vi "Set Image Size.vi"(8 "error in (no error)":errorcluster caption="错误输入（无错误）", 9 "Height":i32, 10 "Width":i32, 11 "ImageListClass 输入":refnum<class "ImageListClass.lvclass"> caption="DNL_LabVIEW Object in") -> (0 "error out":errorcluster caption="错误输出", 3 "ImageListClass 输出":refnum<class "ImageListClass.lvclass"> caption="DNL_LabVIEW Object out")   [LabVIEW 2013, in "ImageListClass.lvclass"]
uses:
  ImageListClass.lvclass
  ImageListClass.lvclass/ImageListClass.ctl
  System.Drawing
  System.Windows.Forms
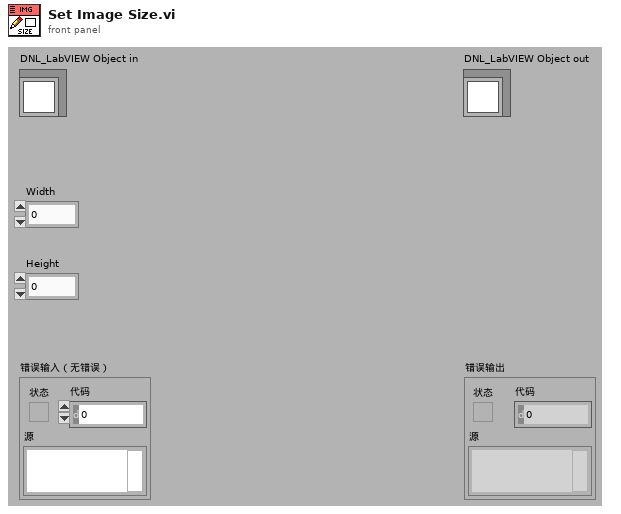
[diagram p1: front panel]
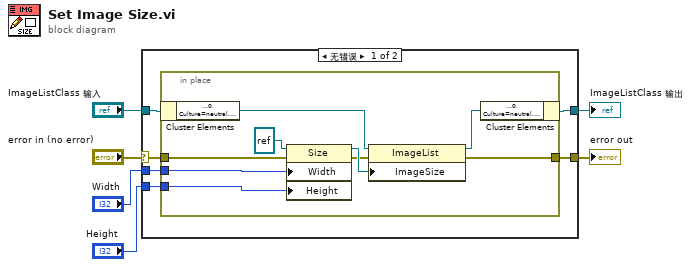
[diagram p0: block diagram]
diagram:
  n1 = case shown="无错误" "error in (no error)" {
    selector: "error in (no error)" -> [w9 w23]
    tunnel: [w8 w23] -> w5
    tunnel: [w7 w22] -> w3
    tunnel: "ImageListClass 输入" -> [w10 w22]
    tunnel: "Width" -> [w12 _]
    tunnel: "Height" -> [w11 _]
    frame No Error {
      n2 = in-place {
        in-place-border: w12 -> [w20]
        in-place-border: w11 -> [w19]
        in-place-border: w9 -> [w16]
        in-place-border: [w14] -> w8
        n3 = in-place-cluster #1(w10) -> ("ImageList"=w18:refnum<k24>)
        n4 = property class="Size"(reference=refnum<k24> refnum ("引用"), error in=w16, "Width"=w20, "Height"=w19) -> (reference out=w21:refnum<k24>, error out=w15:errorcluster)
        n5 = property class="ImageList"(reference=w18, error in=w15, "ImageSize"=w21) -> (reference out=w17:refnum<k24>, error out=w14:errorcluster)
        n6 = in-place-cluster #1("ImageList"=w17) -> (w7:refnum<class "ImageListClass.lvclass">)
      }
    }
    frame Error {
    }
  }
  "error out" <- w5
  "ImageListClass 输出" <- w3
